vi "多帧接收机制(EV05).vi"(0 "can卡类型":u8, 1 "设备索引号":u8, 2 "CAN端口":u8, 3 "VCI_Receive":T1 {"Rsv3" max=0 format="%x"; "Rsv2" min=101 format="%x"; "Rsv1" format="%x"; "Data8" format="%x"; "Data7" format="%x"; "Data6" format="%x"; "Data5" format="%x"; "Data4" format="%x"; "Data3" format="%x"; "Data2" format="%x"; "Data1" format="%x"; "DataLen" format="%x"; "ExternFlag" format="%x"; "RemoteFlag" format="%x"; "SendType" format="%x"; "TimeFlag" format="%x"; "TimeStamp" format="%x"; "ID" format="%x"}, 4 "命令":u32 format="%x", 5 "板号":u32 format="%x", 6 "流控帧":refnum<vi>, 7 "写?":bool, 8 "流控帧2":refnum<vi>, 9 "命令序号":u8) -> (13 "错误信号":bool, 14 "错误代码":i32, 15 "多帧数据长度":i32, 16 "命令序号":u8, 17 "输出数组":u8[](array[numeric]), 18 "读错误代码":u8[](array[numeric]), 19 "结束信号":bool)   [LabVIEW 2013]
panel:
  in  "最大帧号":i32
  out "多帧个数":i32
  out "长度1":i32
  out "接收完成":bool
  in  "多帧计时":bool
  in  "Reset 2":bool caption="重置"
  in  "Reset":bool caption="重置"
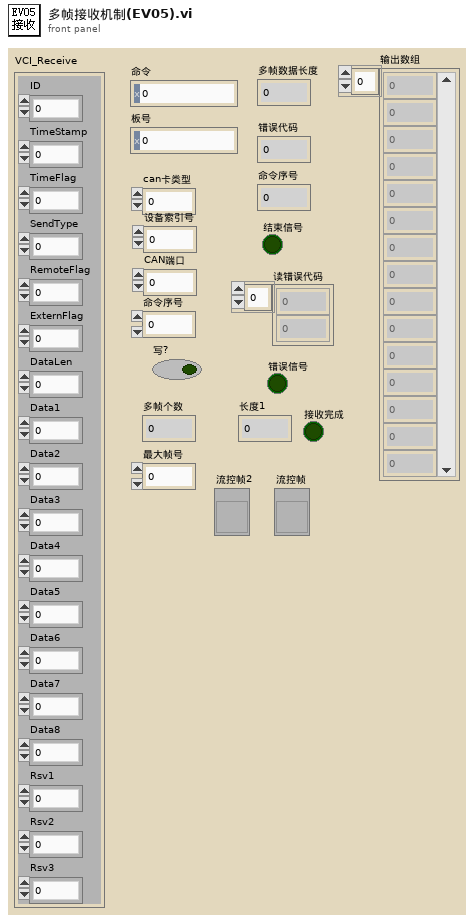
[diagram p1: front panel]
types:
  T1 = cluster{"ID":u32, "TimeStamp":u32, "TimeFlag":u8, "SendType":u8, "RemoteFlag":u8, "ExternFlag":u8, "DataLen":u8, "Data1":u8, "Data2":u8, "Data3":u8, "Data4":u8, "Data5":u8, "Data6":u8, "Data7":u8, "Data8":u8, "Rsv1":u8, "Rsv2":u8, "Rsv3":u8}
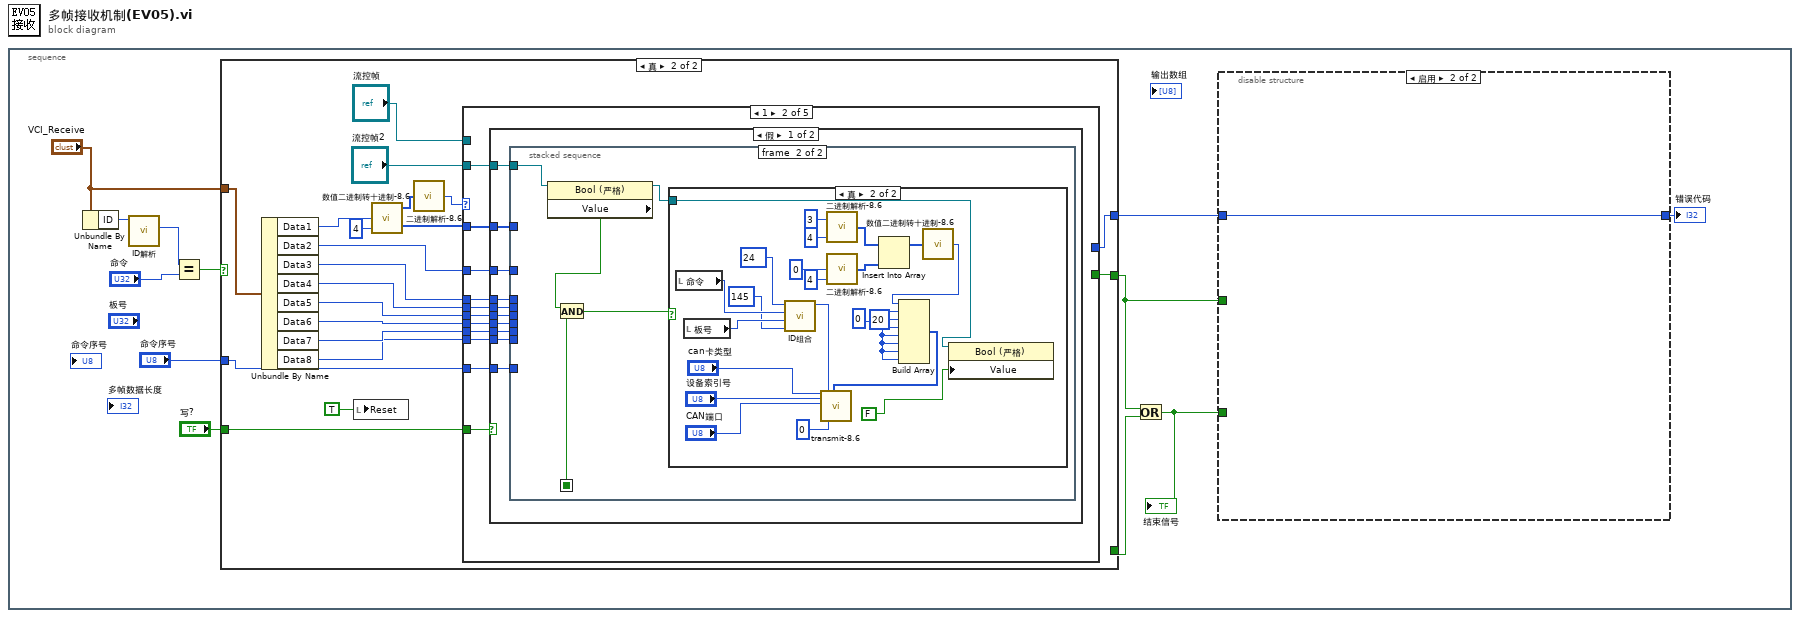
[diagram p0: block diagram]
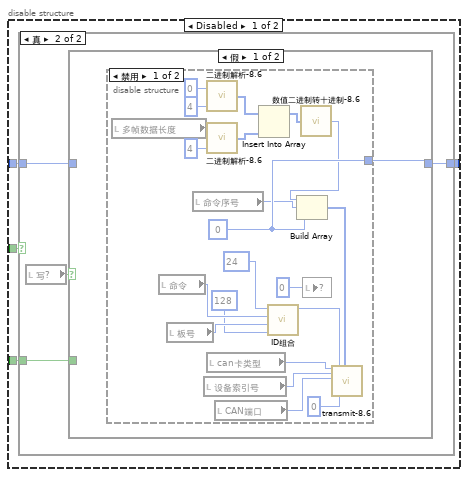
[diagram p2: hidden frame]
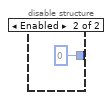
[diagram p4: hidden frame]
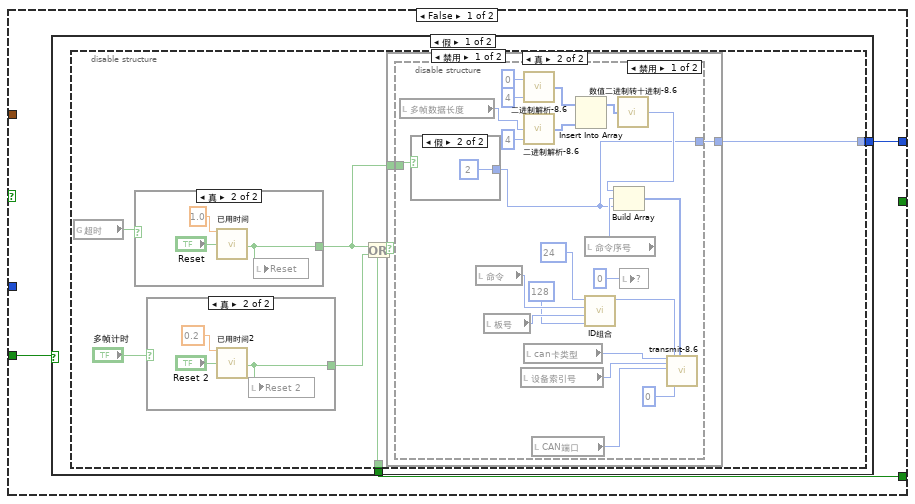
[diagram p6: hidden frame]
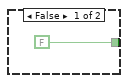
[diagram p8: hidden frame]
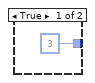
[diagram p10: hidden frame]
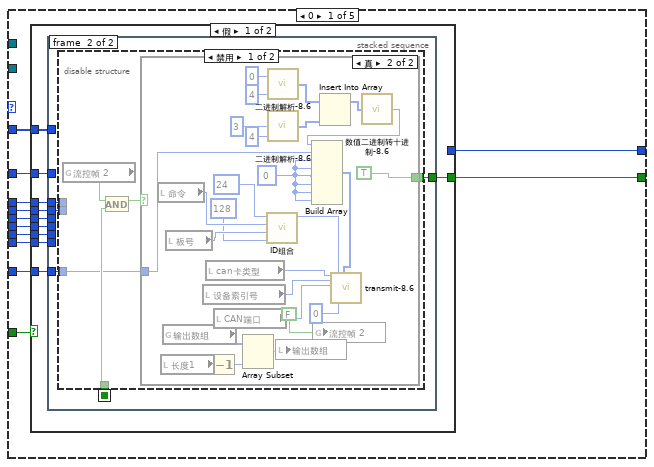
[diagram p14: hidden frame]
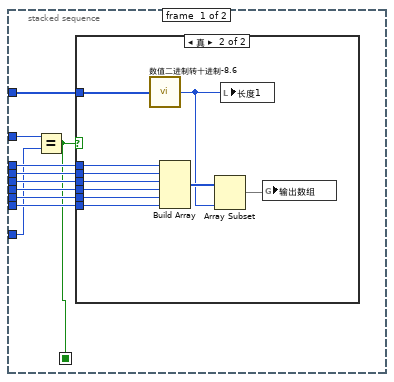
[diagram p15: hidden frame]
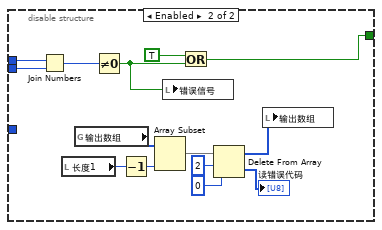
[diagram p18: hidden frame]
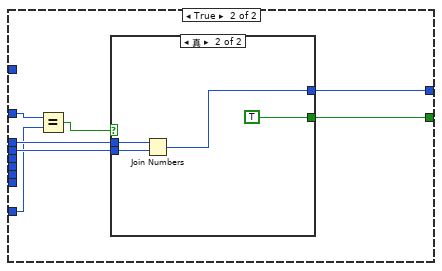
[diagram p19: hidden frame]
diagram:
  n1 = stacked-sequence {
    frame #0 {
      n2 = Unbundle By Name("VCI_Receive") -> ("ID"=w12:u32)
      n3 = call "ID解析.vi"("ID"=w12) -> ("PF(2)"=w11:i32)  [unwired: 10 out]
      n4 = Equal?(x=w11, y="命令") -> (x = y?=w5:bool)
      n5 = case shown="真" w5 {
        tunnel: "VCI_Receive" -> [_ w110]
        tunnel: [_ w96] -> w8
        tunnel: [w49 _] -> w4
        tunnel: [w48 w95] -> w7
        tunnel: "写?" -> [w47 w94]
        tunnel: "命令序号" -> [_ w93]
        frame False {
          n6 = case shown="假" w47 {
            tunnel: [w51 _] -> w49
            tunnel: [w50 _] -> w48
            frame False {
              n7 = disable-structure shown="禁用" {
                disable-tunnel: [w54 _] -> w51
                disable-tunnel: [w53 _] -> w50
                frame Disabled {
                  n8 = global read "EV05全局变量1.vi" "超时"() -> (w52:bool)
                  n9 = case shown="真" w52 {
                    tunnel: [_ w60] -> w56
                    frame False {
                    }
                    frame True {
                      n10 = call "已用时间"("Time Target (s)"=1.0, "Reset"="Reset") -> ("Time has Elapsed"=w60:bool)  [unwired: 3 in, 14 out]
                      n11 = local write "Reset"(w60) -> ()
                    }
                  }
                  n12 = case shown="真" "多帧计时" {
                    tunnel: [FALSE ("Time has Elapsed") w62] -> w55
                    frame False {
                    }
                    frame True {
                      n13 = call "已用时间2"("Time Target (s)"=0.2, "Reset"="Reset 2") -> ("Time has Elapsed"=w62:bool)  [unwired: 3 in, 14 out]
                      n14 = local write "Reset 2"(w62) -> ()
                    }
                  }
                  n15 = Or(x=w56, y=w55) -> (x .or. y?=w54:bool)
                  n16 = case shown="真" w54 {
                    tunnel: w56 -> [_ w66]
                    tunnel: [_ w65] -> w53
                    frame False {
                    }
                    frame True {
                      n17 = disable-structure shown="禁用" {
                        disable-tunnel: w66 -> [w81 _]
                        disable-tunnel: [w70 _] -> w65
                        frame Disabled {
                          n18 = local read "多帧数据长度"() -> (w72:i32)
                          n19 = case shown="假" w81 {
                            tunnel: [3 ("元素") 2 ("元素")] -> w70
                            frame True {
                            }
                            frame False {
                            }
                          }
                          n20 = local read "命令"() -> (w84:u32)
                          n21 = local read "板号"() -> (w69:u32)
                          n22 = local read "设备索引号"() -> (w87:u8)
                          n23 = call "二进制解析-8.6.vi"("索引"=4, "数值"=0) -> ("低位子数组"=w75:i32[])  [unwired: 3 out]
                          n24 = call "二进制解析-8.6.vi"("索引"=4, "数值"=w72) -> ("低位子数组"=w74:i32[])  [unwired: 3 out]
                          n25 = local read "can卡类型"() -> (w88:u8)
                          n26 = local read "CAN端口"() -> (w86:u8)
                          n27 = Insert Into Array(array=w75, new element=w74) -> (w73:i32[])  [unwired: 1 in]
                          n28 = local read "命令序号"() -> (w80:u8)
                          n29 = call "ID组合.vi"("SA(4)"=128 ("PDU(1)"), "PS(3)"=w69, "PF(2)"=w84, "PDU(1)"=24) -> ("ID"=w83:i32)  [unwired: 7 out]
                          n30 = call "数值二进制转十进制-8.6.vi"("子数组"=w73) -> ("十进制数值"=w71:i32)  [unwired: 4 out]
                          n31 = Build Array(w71, w80, w70) -> (w82:i32[])
                          n32 = local write item#-1(u8 0 ("计数")) -> ()
                          n33 = call "transmit-8.6.vi"("can卡类型"=w88, "设备索引号"=w87, "CAN端口"=w86, "ID"=w83, "SendType"=u8 0, "Data"=w82) -> ()  [unwired: 3 in, 11 out]
                        }
                        frame Enabled {
                        }
                      }
                    }
                  }
                }
                frame Enabled {
                }
              }
            }
            frame True {
            }
          }
        }
        frame True {
          n34 = Unbundle By Name(w110) -> ("Data1"=w109:u8, "Data2"=w105:u8, "Data3"=w103:u8, "Data4"=w102:u8, "Data5"=w101:u8, "Data6"=w100:u8, "Data7"=w99:u8, "Data8"=w98:u8)
          n35 = local write "Reset"(TRUE ("Reset")) -> ()
          n36 = call "二进制解析-8.6.vi"("索引"=4, "数值"=w109) -> ("低位子数组"=w104:i32[], "高位子数组"=w107:i32[])  [unwired: 2 out]
          n37 = call "数值二进制转十进制-8.6.vi"("子数组"=w107) -> ("十进制数值"=w106:i32)  [unwired: 4 out]
          n38 = case shown="1" w106 {
            tunnel: w105 -> [w122 w224 w314 _ _]
            tunnel: w104 -> [w121 w223 w316 _ _]
            tunnel: w103 -> [w115 w222 w315 _ _]
            tunnel: w102 -> [w120 w221 w313 _ _]
            tunnel: w101 -> [w119 w220 w312 _ _]
            tunnel: w100 -> [w118 w219 w311 _ _]
            tunnel: w99 -> [w117 w218 w310 _ _]
            tunnel: w98 -> [w116 w217 w309 _ _]
            tunnel: [w112 _ w306 _ _] -> w96
            tunnel: [w114 _ _ _ _] -> w95
            tunnel: w94 -> [w113 w216 w305 _ _]
            tunnel: w93 -> [w111 w215 _ _ _]
            tunnel: "流控帧2" -> [_ w214 _ _ _]
            tunnel: "流控帧" -> [_ _ _ w364 _]
            frame 0 {
              n39 = case shown="假" w113 {
                tunnel: w122 -> [w132 w205]
                tunnel: w121 -> [w131 _]
                tunnel: w120 -> [w130 w207]
                tunnel: w119 -> [w129 _]
                tunnel: w118 -> [w128 _]
                tunnel: w117 -> [w127 _]
                tunnel: w116 -> [w126 _]
                tunnel: w115 -> [w125 w208]
                tunnel: [_ w209] -> w114
                tunnel: [w124 w206] -> w112
                tunnel: w111 -> [w123 w204]
                frame False {
                  n40 = stacked-sequence {
                    seq-local: [w133 _] -> [_ w156]
                    tunnel: w132 -> [w135 _]
                    tunnel: w131 -> [w142 _]
                    tunnel: w130 -> [w141 w153]
                    tunnel: w129 -> [w140 _]
                    tunnel: w128 -> [w139 _]
                    tunnel: w127 -> [w138 _]
                    tunnel: w126 -> [w137 _]
                    tunnel: w125 -> [w136 w154]
                    tunnel: [_ w157] -> w124
                    tunnel: w123 -> [w134 w155]
                    frame #0 {
                      n41 = Equal?(x=w135, y=w134) -> (x = y?=w133:bool)
                      n42 = case shown="真" w133 {
                        tunnel: w142 -> [_ w152]
                        tunnel: w141 -> [_ w151]
                        tunnel: w140 -> [_ w150]
                        tunnel: w139 -> [_ w149]
                        tunnel: w138 -> [_ w148]
                        tunnel: w137 -> [_ w147]
                        tunnel: w136 -> [_ w146]
                        frame False {
                        }
                        frame True {
                          n43 = call "数值二进制转十进制-8.6.vi"("子数组"=w152) -> ("十进制数值"=w144:i32)  [unwired: 4 out]
                          n44 = Build Array(w146, w151, w150, w149, w148, w147) -> (w145:u8[])
                          n45 = Array Subset(array=w145, length=w144) -> (w143:u8[])  [unwired: 1 in]
                          n46 = local write "长度1"(w144) -> ()
                          n47 = global write "EV05全局变量1.vi" "输出数组"(w143) -> ()
                        }
                      }
                    }
                    frame #1 {
                      n48 = disable-structure shown="禁用" {
                        disable-tunnel: [w162 w191] -> w157
                        disable-tunnel: w156 -> [w161 _]
                        disable-tunnel: w155 -> [w158 _]
                        disable-tunnel: w154 -> [_ w197]
                        disable-tunnel: w153 -> [_ w198]
                        frame Disabled {
                          n49 = global read "EV05全局变量1.vi" "流控帧 2"() -> (w159:bool)
                          n50 = And(x=w159, y=w161) -> (x .and. y?=w160:bool)
                          n51 = case shown="真" w160 {
                            tunnel: [_ TRUE] -> w162
                            tunnel: w158 -> [_ w165]
                            frame False {
                            }
                            frame True {
                              w181 = 0 ("元素")
                              n52 = local read "命令"() -> (w184:u32)
                              n53 = local read "长度1"() -> (w167:i32)
                              n54 = global read "EV05全局变量1.vi" "输出数组"() -> (w169:u8[])
                              n55 = local read "板号"() -> (w173:u32)
                              n56 = local read "设备索引号"() -> (w187:u8)
                              n57 = local read "can卡类型"() -> (w188:u8)
                              n58 = Decrement(x=w167) -> (x-1=w166:i32)
                              n59 = local read "CAN端口"() -> (w186:u8)
                              n60 = Array Subset(array=w169, length=w166) -> (w168:u8[])  [unwired: 1 in]
                              n61 = call "ID组合.vi"("SA(4)"=128 ("PDU(1)"), "PS(3)"=w173, "PF(2)"=w184, "PDU(1)"=24) -> ("ID"=w183:i32)  [unwired: 7 out]
                              n62 = call "二进制解析-8.6.vi"("索引"=4, "数值"=0) -> ("低位子数组"=w177:i32[])  [unwired: 3 out]
                              n63 = call "二进制解析-8.6.vi"("索引"=4, "数值"=3) -> ("低位子数组"=w174:i32[])  [unwired: 3 out]
                              n64 = local write "输出数组"(w168) -> ()
                              n65 = global write "EV05全局变量1.vi" "流控帧 2"(FALSE ("流控帧 2")) -> ()
                              n66 = Insert Into Array(array=w177, new element=w174) -> (w176:i32[])  [unwired: 1 in]
                              n67 = call "数值二进制转十进制-8.6.vi"("子数组"=w176) -> ("十进制数值"=w175:i32)  [unwired: 4 out]
                              n68 = Build Array(w175, w165, w181, w181, w181, w181, w181, w181) -> (w182:i32[])
                              n69 = call "transmit-8.6.vi"("can卡类型"=w188, "设备索引号"=w187, "CAN端口"=w186, "ID"=w183, "SendType"=u8 0, "Data"=w182) -> ()  [unwired: 3 in, 11 out]
                            }
                          }
                        }
                        frame Enabled {
                          n70 = Join Numbers(hi=w197, lo=w198) -> ((hi.lo)=w196:u16)
                          n71 = local read "长度1"() -> (w200:i32)
                          n72 = global read "EV05全局变量1.vi" "输出数组"() -> (w202:u8[])
                          n73 = Not Equal To 0?(x=w196) -> (x != 0?=w189:bool)
                          n74 = Decrement(x=w200) -> (x-1=w199:i32)
                          n75 = Array Subset(array=w202, length=w199) -> (w201:u8[])  [unwired: 1 in]
                          n76 = local write "错误信号"(w189) -> ()
                          n77 = Or(x=TRUE, y=w189) -> (x .or. y?=w191:bool)
                          n78 = Delete From Array(array=w201, length=2 ("长度"), index=0 ("索引")) -> (deleted portion=→"读错误代码":u8[], array with subset deleted=w195:u8[])
                          n79 = local write "输出数组"(w195) -> ()
                        }
                      }
                    }
                  }
                }
                frame True {
                  n80 = Equal?(x=w205, y=w204) -> (x = y?=w203:bool)
                  n81 = case shown="真" w203 {
                    tunnel: [_ w213] -> w209
                    tunnel: w208 -> [_ w212]
                    tunnel: w207 -> [_ w211]
                    tunnel: [_ TRUE] -> w206
                    frame False {
                    }
                    frame True {
                      n82 = Join Numbers(hi=w212, lo=w211) -> ((hi.lo)=w213:u16)
                    }
                  }
                }
              }
            }
            frame 1 {
              n83 = case shown="假" w216 {
                tunnel: w224 -> [w234 _]
                tunnel: w223 -> [w233 _]
                tunnel: w222 -> [w232 _]
                tunnel: w221 -> [w231 _]
                tunnel: w220 -> [w230 _]
                tunnel: w219 -> [w229 _]
                tunnel: w218 -> [w228 _]
                tunnel: w217 -> [w227 _]
                tunnel: w215 -> [w226 _]
                tunnel: w214 -> [w225 _]
                frame False {
                  n84 = stacked-sequence {
                    seq-local: [w235 _] -> [_ w282]
                    tunnel: w234 -> [w244 _]
                    tunnel: w233 -> [w243 _]
                    tunnel: w232 -> [w237 _]
                    tunnel: w231 -> [w242 _]
                    tunnel: w230 -> [w241 _]
                    tunnel: w229 -> [w240 _]
                    tunnel: w228 -> [w239 _]
                    tunnel: w227 -> [w238 _]
                    tunnel: w226 -> [w236 _]
                    tunnel: w225 -> [_ w280]
                    frame #0 {
                      n85 = Equal?(x=w237, y=w236) -> (x = y?=w235:bool)
                      n86 = case shown="真" w235 {
                        tunnel: w244 -> [_ w251]
                        tunnel: w243 -> [_ w250]
                        tunnel: w242 -> [_ w249]
                        tunnel: w241 -> [_ w248]
                        tunnel: w240 -> [_ w247]
                        tunnel: w239 -> [_ w246]
                        tunnel: w238 -> [_ w245]
                        frame False {
                        }
                        frame True {
                          n87 = stacked-sequence {
                            tunnel: w251 -> [w265 _]
                            tunnel: w250 -> [w263 _]
                            tunnel: w249 -> [_ w277]
                            tunnel: w248 -> [_ w276]
                            tunnel: w247 -> [_ w275]
                            tunnel: w246 -> [_ w274]
                            tunnel: w245 -> [_ w273]
                            frame #0 {
                              n88 = call "二进制解析-8.6.vi"("索引"=8, "数值"=w265) -> ("低位子数组"=w264:i32[])  [unwired: 3 out]
                              n89 = Insert Into Array(array=w263, new element=w264) -> (w262:i32[])  [unwired: 1 in]
                              n90 = call "数值二进制转十进制-8.6.vi"("子数组"=w262) -> ("十进制数值"=w260:i32)  [unwired: 4 out]
                              "长度1" <- w260
                              n91 = for {
                                N: w260 -> [_]
                                tunnel: [u8 0] -> w261 mode=indexing
                              }
                              n92 = Subtract(x=w260, y=6) -> (x-y=w258:i32)
                              n93 = global write "EV05全局变量1.vi" "输出数组"(w261) -> ()
                              n94 = Quotient & Remainder(x=w258, y=7) -> (x-y*floor(x/y)=w256:i32, floor(x/y)=w254:i32)
                              n95 = Equal To 0?(x=w256) -> (x = 0?=w255:bool)
                              n96 = Increment(x=w254) -> (x+1=w253:i32)
                              n97 = Select(t=w254, s=w255, f=w253) -> (s? t:f=→"多帧个数":i32)
                            }
                            frame #1 {
                              n98 = Build Array(w277, w276, w275, w274, w273) -> (w271:u8[])
                              n99 = global read "EV05全局变量1.vi" "输出数组"() -> (w272:u8[])
                              n100 = local write "最大帧号"(1 ("最大帧号")) -> ()
                              n101 = Replace Array Subset(array=w272, new element=w271, index=0 ("索引")) -> (w270:u8[])
                              n102 = global write "EV05全局变量1.vi" "输出数组"(w270) -> ()
                            }
                          }
                        }
                      }
                    }
                    frame #1 {
                      n103 = property class="Bool (严格)"(reference=w280) -> (reference out=w278:refnum<vi>, "Value"=w279:bool)  [unwired: 1 in, 1 out]
                      n104 = And(x=w279, y=w282) -> (x .and. y?=w281:bool)
                      n105 = case shown="真" w281 {
                        tunnel: w278 -> [_ w284]
                        frame False {
                        }
                        frame True {
                          w290 = 0 ("元素")
                          n106 = local read "命令"() -> (w291:u32)
                          n107 = local read "板号"() -> (w287:u32)
                          n108 = call "ID组合.vi"("SA(4)"=145 ("PDU(1)"), "PS(3)"=w287, "PF(2)"=w291, "PDU(1)"=24) -> ("ID"=w293:i32)  [unwired: 7 out]
                          n109 = call "二进制解析-8.6.vi"("索引"=4, "数值"=3) -> ("低位子数组"=w298:i32[])  [unwired: 3 out]
                          n110 = call "二进制解析-8.6.vi"("索引"=4, "数值"=0) -> ("低位子数组"=w297:i32[])  [unwired: 3 out]
                          n111 = Insert Into Array(array=w298, new element=w297) -> (w296:i32[])  [unwired: 1 in]
                          n112 = call "数值二进制转十进制-8.6.vi"("子数组"=w296) -> ("十进制数值"=w295:i32)  [unwired: 4 out]
                          n113 = Build Array(w295, w290, 20 ("元素"), w290, w290, w290, w290, w290) -> (w294:i32[])
                          n114 = call "transmit-8.6.vi"("can卡类型"="can卡类型", "设备索引号"="设备索引号", "CAN端口"="CAN端口", "ID"=w293, "SendType"=u8 0, "Data"=w294) -> ()  [unwired: 3 in, 11 out]
                          n115 = property class="Bool (严格)"(reference=w284, "Value"=FALSE ("流控")) -> ()  [unwired: 1 in, 2 out]
                        }
                      }
                    }
                  }
                }
                frame True {
                }
              }
            }
            frame 2 {
              n116 = case shown="假" w305 {
                tunnel: w316 -> [w325 _]
                tunnel: w315 -> [w324 _]
                tunnel: w314 -> [w323 _]
                tunnel: w313 -> [w322 _]
                tunnel: w312 -> [w321 _]
                tunnel: w311 -> [w320 _]
                tunnel: w310 -> [w319 _]
                tunnel: w309 -> [w318 _]
                tunnel: [w317 _] -> w306
                frame False {
                  n117 = stacked-sequence {
                    seq-local: [w327 _] -> [_ w345]
                    seq-local: [w326 _] -> [_ w347]
                    tunnel: w325 -> [w344 _]
                    tunnel: w324 -> [w343 _]
                    tunnel: w323 -> [w342 _]
                    tunnel: w322 -> [w341 _]
                    tunnel: w321 -> [w340 _]
                    tunnel: w320 -> [w339 _]
                    tunnel: w319 -> [w338 _]
                    tunnel: w318 -> [w337 _]
                    tunnel: [_ w361] -> w317
                    frame #0 {
                      n118 = call "数值二进制转十进制-8.6.vi"("子数组"=w344) -> ("十进制数值"=w329:i32)  [unwired: 4 out]
                      n119 = Build Array(w342, w343, w341, w340, w339, w338, w337) -> (w330:u8[])
                      n120 = Decrement(x=w329) -> (x-1=w334:i32)
                      n121 = Multiply(x=w334, y=7) -> (x*y=w333:i32)
                      n122 = Max & Min(x="最大帧号", y=w329) -> (max(x,y)=w327:i32)  [unwired: 1 out]
                      n123 = Add(x=w333, y=5) -> (x+y=w331:i32)
                      n124 = global read "EV05全局变量1.vi" "输出数组"() -> (w336:u8[])
                      n125 = Replace Array Subset(array=w336, new element=w330, index=w331) -> (w326:u8[])
                      n126 = local write "最大帧号"(w327) -> ()
                      n127 = global write "EV05全局变量1.vi" "输出数组"(w326) -> ()
                    }
                    frame #1 {
                      n128 = local read "长度1"() -> (w359:i32)
                      n129 = local read "多帧个数"() -> (w346:i32)
                      n130 = Decrement(x=w359) -> (x-1=w358:i32)
                      n131 = Array Subset(array=w347, length=w358) -> (w360:u8[])  [unwired: 1 in]
                      n132 = Equal?(x=w345, y=w346) -> (x = y?=w362:bool)
                      "接收完成" <- w362
                      n133 = Delete From Array(array=w360, length=2 ("长度"), index=0 ("索引")) -> (deleted portion=w354:u8[], array with subset deleted=w357:u8[])
                      n134 = local write "读错误代码"(w354) -> ()
                      n135 = Index Array(array=w354, index #1=0 ("索引"), index #2=1 ("索引")) -> (element #1=w350:u8, element #2=w351:u8)
                      n136 = local write "输出数组"(w357) -> ()
                      n137 = Join Numbers(hi=w350, lo=w351) -> ((hi.lo)=w349:u16)
                      n138 = Not Equal To 0?(x=w349) -> (x != 0?=w348:bool)
                      "错误信号" <- w348
                      n139 = Or(x=w362, y=w348) -> (x .or. y?=w361:bool)
                    }
                  }
                }
                frame True {
                }
              }
              n140 = local write "多帧计时"(TRUE ("多帧计时")) -> ()
              n141 = local write "Reset 2"(TRUE ("Reset 2")) -> ()
            }
            frame 3 {
              n142 = disable-structure shown="禁用" {
                frame Disabled {
                  n143 = global write "EV05全局变量1.vi" "流控帧"(TRUE ("Reset")) -> ()
                }
                frame Enabled {
                }
              }
              n144 = property class="Bool (严格)"(reference=w364, "Value"=TRUE ("值")) -> ()  [unwired: 1 in, 2 out]
            }
            frame 4, Default {
            }
          }
        }
      }
      n145 = Or(x=w8, y=w4) -> (x .or. y?=w2:bool)
      "结束信号" <- w2
      n146 = disable-structure shown="启用" {
        disable-tunnel: w8 -> [w16 _]
        disable-tunnel: w7 -> [w15 w46]
        disable-tunnel: [w14 w46] -> w6
        disable-tunnel: w2 -> [w13 _]
        frame Disabled {
          n147 = case shown="真" w16 {
            tunnel: w15 -> [w17 w19]
            tunnel: [w17 w21] -> w14
            tunnel: w13 -> [_ w18]
            frame False {
            }
            frame True {
              n148 = local read "写?"() -> (w20:bool)
              n149 = case shown="假" w20 {
                tunnel: [w22 w45] -> w21
                tunnel: w19 -> [_ w45]
                tunnel: w18 -> [_ _]
                frame False {
                  n150 = disable-structure shown="禁用" {
                    disable-tunnel: [w43 0 ("元素")] -> w22
                    frame Disabled {
                      w43 = 0 ("元素")
                      n151 = local read "多帧数据长度"() -> (w41:i32)
                      n152 = local read "命令"() -> (w30:u32)
                      n153 = local read "板号"() -> (w25:u32)
                      n154 = local read "命令序号"() -> (w33:u8)
                      n155 = local read "设备索引号"() -> (w27:u8)
                      n156 = call "二进制解析-8.6.vi"("索引"=4, "数值"=0) -> ("低位子数组"=w38:i32[])  [unwired: 3 out]
                      n157 = call "二进制解析-8.6.vi"("索引"=4, "数值"=w41) -> ("低位子数组"=w39:i32[])  [unwired: 3 out]
                      n158 = local read "can卡类型"() -> (w26:u8)
                      n159 = local read "CAN端口"() -> (w28:u8)
                      n160 = Insert Into Array(array=w38, new element=w39) -> (w40:i32[])  [unwired: 1 in]
                      n161 = call "ID组合.vi"("SA(4)"=128 ("PDU(1)"), "PS(3)"=w25, "PF(2)"=w30, "PDU(1)"=24) -> ("ID"=w31:i32)  [unwired: 7 out]
                      n162 = call "数值二进制转十进制-8.6.vi"("子数组"=w40) -> ("十进制数值"=w42:i32)  [unwired: 4 out]
                      n163 = Build Array(w42, w33, w43) -> (w32:i32[])
                      n164 = local write item#-1(u8 0 ("计数")) -> ()
                      n165 = call "transmit-8.6.vi"("can卡类型"=w26, "设备索引号"=w27, "CAN端口"=w28, "ID"=w31, "SendType"=u8 0, "Data"=w32) -> ()  [unwired: 3 in, 11 out]
                    }
                    frame Enabled {
                    }
                  }
                }
                frame True {
                }
              }
            }
          }
        }
        frame Enabled {
        }
      }
      "错误代码" <- w6
    }
  }
